vi "WFGetDtFs.vi"   [LabVIEW 2013]
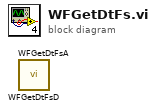
[diagram p0: block diagram]
diagram:
  n1 = call "WFGetDtFsD.vi"() -> ()  [unwired: 10 in, 2 out]
  n2 = call "WFGetDtFsA.vi"() -> ()  [unwired: 10 in, 2 out]
